vi "TDTRX6-Write Output Buffers.vi"(0 "RPcox":refnum<k7>, 5 "Next Buffer":i32, 7 "Input array":dbl[][](array[numeric]), 9 "Chans":i32[](array[numeric]), 11 "error in (no error)":errorcluster) -> (15 "error out":errorcluster)   [LabVIEW 2015]
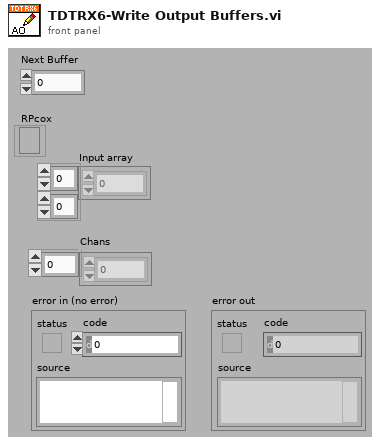
[diagram p1: front panel]
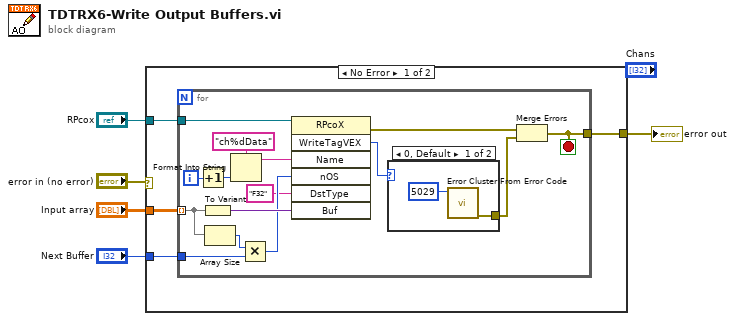
[diagram p0: block diagram]
diagram:
  n1 = case shown="No Error" "error in (no error)" {
    selector: "error in (no error)" -> [_ w27]
    tunnel: "Next Buffer" -> [w9 _]
    tunnel: "Input array" -> [w8 _]
    tunnel: "RPcox" -> [w7 _]
    tunnel: [w6 w27] -> w1
    frame No Error {
      n2 = for {
        tunnel: w7 -> [w24]
        tunnel: w8 -> [w13] mode=indexing
        tunnel: [w11] -> w6
        tunnel: w9 -> [w18]
        i -> [w21]
        stop <- w11 stop-if-true
        n3 = Increment(x=w21) -> (x+1=w22:i32)
        n4 = To Variant(anything=w13) -> (Variant=w17:variant)
        n5 = Array Size(array=w13) -> (size(s)=w14:i32)
        n6 = Format Into String(format string="ch%dData", w22) -> (resulting string=w20:string)  [unwired: 2 in, 1 out]
        n7 = Multiply(x=w14, y=w18) -> (x*y=w16:i32)
        n8 = invoke class="RPcoX" method="WriteTagVEX"(reference=w24, "Name"=w20, "nOS"=w16, "DstType"="F32", "Buf"=w17) -> (error out=w19:errorcluster, "WriteTagVEX"=w12:i32)  [unwired: 2 in, 5 out]
        n9 = case shown="0, Default" w12 {
          tunnel: [w25 _] -> w10
          frame 0, Default {
            n10 = call <vilib>:"Error Cluster From Error Code.vi"("error code (0)"=5029) -> ("error out"=w25:errorcluster)  [unwired: 8 in]
          }
          frame 1 {
          }
        }
        n11 = Merge Errors(w19, w10) -> (w11:errorcluster)
      }
    }
    frame Error {
    }
  }
  "error out" <- w1
